vi "Calibration - Config (SubVI).vi"(7 "Action":enum16{"Save", "Load"}(ring)=enum."Load", 8 "error in (no error)":errorcluster, 10 "Path":path, 11 "DS":T2) -> (0 "error out":errorcluster, 3 "DS out":T2={"Timeout"=-1, "LC MC"=[], "TD MC"=[], "Motor Pulse"=0, "Disp M"=[], "LC Unit"=[], "Disp Unit"=[], "TD Unit"=[], "LC Name"=[], "TD Name"=[], "Machine"=enum."Please Select", "Sensor Port"=[]})   [LabVIEW 2019]
uses:
  Controls/Calibration - Data Structure.ctl
  <vilib>/Utility/config.llb/Write Key (String).vi
  <vilib>/Utility/config.llb/Write Key (Double).vi
  <vilib>/Utility/config.llb/Read Key (String).vi
  <vilib>/Utility/config.llb/Read Key (Double).vi
  <vilib>/Utility/config.llb/NI_LVConfig.lvlib
panel:
  in  "Sensor Port":T1(ring)
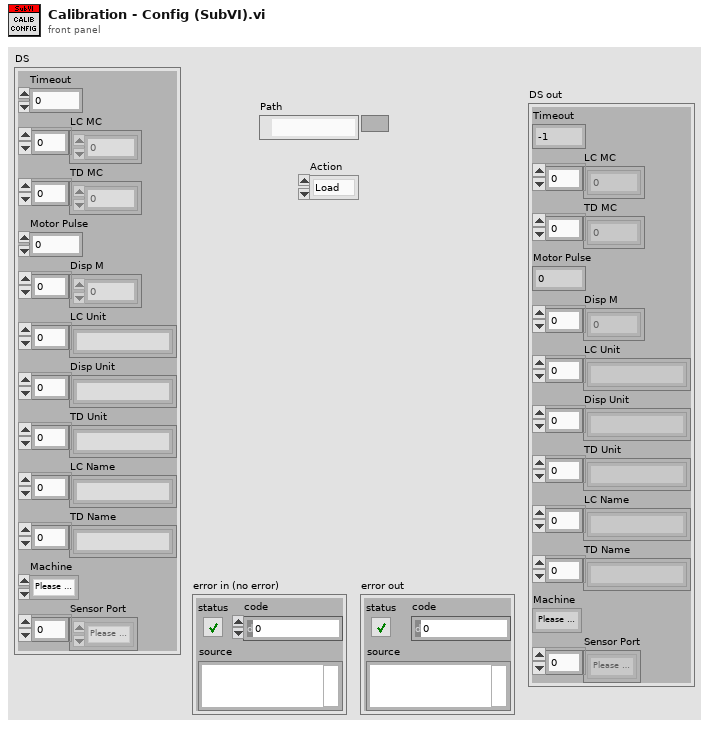
[diagram p1: front panel]
types:
  T1 = enum16{"Please Select", "LC 1", "LC 2", "LC 3", "LC 4", "LC 5", "LC 6", "LC 7", "LC 8", "TD 1", "TD 2", "TD 3", "TD 4", "TD 5", "TD 6", "TD 7", "TD 8", "TD 9", "TD 10", "TD 11", "TD 12"}
  T2 = typedef "Calibration - Data Structure.ctl" = cluster{"Timeout":i32, "LC MC":dbl[], "TD MC":dbl[], "Motor Pulse":u64, "Disp M":dbl[], "LC Unit":string[], "Disp Unit":string[], "TD Unit":string[], "LC Name":string[], "TD Name":string[], "Machine":enum16{"Please Select", "Motor 1", "Motor 2", "Motor 3", "Motor 4", "Motor 5", "Motor 6", "Motor 7", "Motor 8", "Motor 9"}, "Sensor Port":enum16{"Please Select", "LC 1", "LC 2", "LC 3", "LC 4", "LC 5", "LC 6", "LC 7", "LC 8", "TD 1", "TD 2", "TD 3", "TD 4", "TD 5", "TD 6", "TD 7", "TD 8", "TD 9", "TD 10", "TD 11", "TD 12"}[]}
  T3 = typedef "NI_LVConfig.lvlib/Config Data RefNum.ctl" = refnum<k1>
  T4 = enum16{"Please Select", "LC 1", "LC 2", "LC 3", "LC 4", "LC 5", "LC 6", "LC 7", "LC 8", "TD 1", "TD 2", "TD 3", "TD 4", "TD 5", "TD 6", "TD 7", "TD 8", "TD 9", "TD 10", "TD 11", "TD 12"}[]
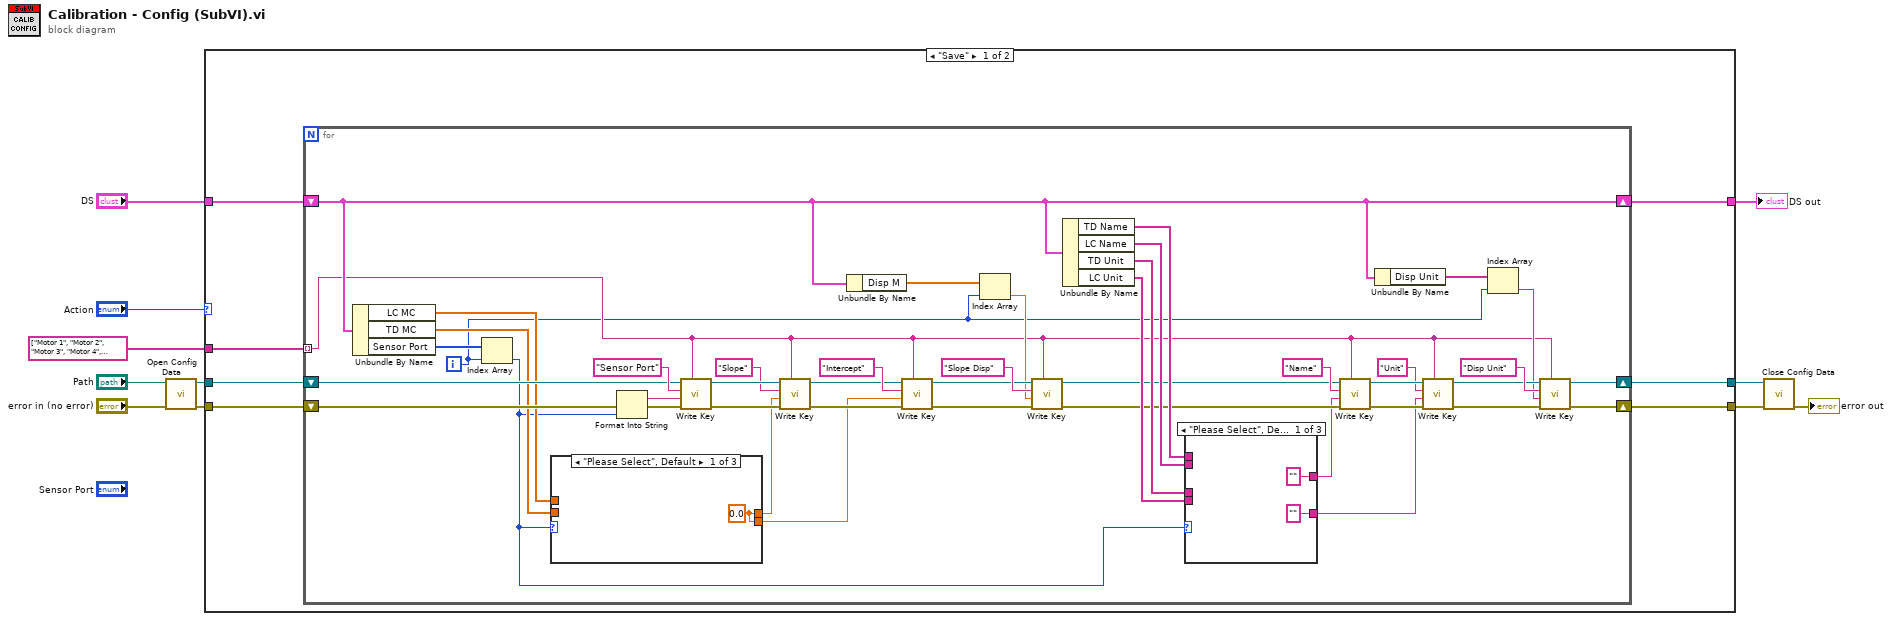
[diagram p0: block diagram]
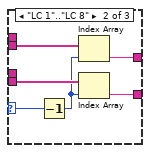
[diagram p2: hidden frame]
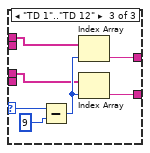
[diagram p3: hidden frame]
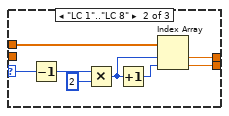
[diagram p4: hidden frame]
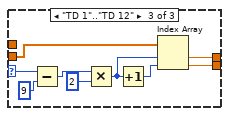
[diagram p5: hidden frame]
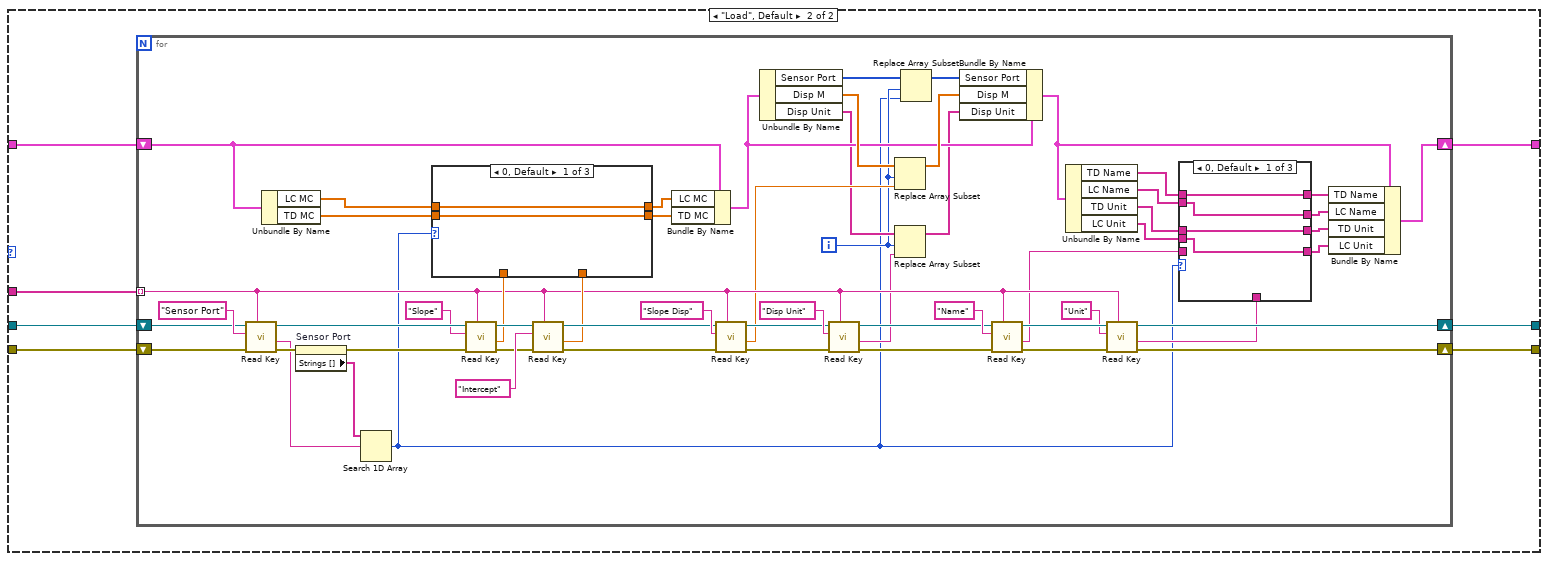
[diagram p6: hidden frame]
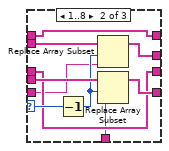
[diagram p7: hidden frame]
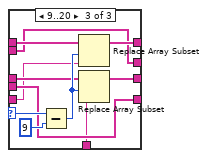
[diagram p8: hidden frame]
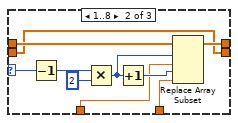
[diagram p9: hidden frame]
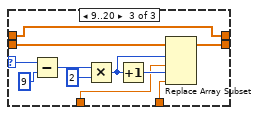
[diagram p10: hidden frame]
diagram:
  n1 = call <vilib>:"Open Config Data.vi"("error in (no error)"="error in (no error)", "configuration file path"="Path") -> ("error out"=w4:errorcluster, "refnum"=w7:T3)  [unwired: 7 in, 1 out]
  n2 = case shown="\"Save\"" "Action" {
    tunnel: "DS" -> [w16 w97]
    tunnel: [w14 w100] -> w9
    tunnel: [w15 w101] -> w8
    tunnel: w7 -> [w17 w102]
    tunnel: w4 -> [w18 w99]
    tunnel: [w13 w98] -> w2
    tunnel: string[] ["Motor 1", "Motor 2", "Motor 3", "Motor 4", "Motor 5", "Motor 6", "Motor 7", "Motor 8", "Motor 9"] ("Strings []") -> [w12 w96]
    frame "Save" {
      n3 = for {
        shift-right: [w22] -> w14
        shift-left: w18 -> [w61]
        shift-right: [w23] -> w15
        shift-left: w17 -> [w58]
        shift-right: [w21] -> w13
        shift-left: w16 -> [w21]
        tunnel: w12 -> [w20] mode=indexing
        i -> [w19]
        n4 = Unbundle By Name(w21) -> ("LC MC"=w50:dbl[], "TD MC"=w51:dbl[], "Sensor Port"=w42:T4)
        n5 = Index Array(array=w42, index=w19) -> (element=w41:T1)
        n6 = case shown="\"Please Select\", Default" w41 {
          selector: w41 -> [_ w85 w90]
          tunnel: w51 -> [_ _ w87]
          tunnel: w50 -> [_ w86 _]
          tunnel: [w78 w80 w92] -> w49
          tunnel: [w78 w79 w91] -> w48
          frame "Please Select", Default {
            w78 = 0.0 ("Numeric")
          }
          frame "LC 1".."LC 8" {
            n7 = Decrement(x=w85) -> (x-1=w83:T1)
            n8 = Multiply(x=w83, y=2) -> (x*y=w81:i32)
            n9 = Increment(x=w81) -> (x+1=w82:i32)
            n10 = Index Array(array=w86, index #1=w81, index #2=w82) -> (element #1=w80:dbl, element #2=w79:dbl)
          }
          frame "TD 1".."TD 12" {
            n11 = Subtract(x=w90, y=9) -> (x-y=w89:i32)
            n12 = Multiply(x=w89, y=2) -> (x*y=w93:i32)
            n13 = Increment(x=w93) -> (x+1=w94:i32)
            n14 = Index Array(array=w87, index #1=w93, index #2=w94) -> (element #1=w92:dbl, element #2=w91:dbl)
          }
        }
        n15 = Format Into String(error in=w61, w41) -> (resulting string=w60:string, error out=w59:errorcluster)  [unwired: 2 in]
        n16 = call-poly <vilib>:"Write Key.vi"("section"=w20, "error in (no error)"=w59, "value"=w60, "key"="Sensor Port" ("section"), "refnum"=w58) -> ("error out"=w57:errorcluster, "refnum out"=w56:T3)  [unwired: 4 in, 1 out]
        n17 = call-poly <vilib>:"Write Key.vi"("section"=w20, "error in (no error)"=w57, "value"=w49, "key"="Slope" ("section"), "refnum"=w56) -> ("error out"=w53:errorcluster, "refnum out"=w52:T3)  [unwired: 4 in, 1 out]
        n18 = Unbundle By Name(w21) -> ("Disp M"=w44:dbl[])
        n19 = call-poly <vilib>:"Write Key.vi"("section"=w20, "error in (no error)"=w53, "value"=w48, "key"="Intercept" ("section"), "refnum"=w52) -> ("error out"=w46:errorcluster, "refnum out"=w45:T3)  [unwired: 4 in, 1 out]
        n20 = Index Array(array=w44, index=w19) -> (element=w43:dbl)
        n21 = call-poly <vilib>:"Write Key.vi"("section"=w20, "error in (no error)"=w46, "value"=w43, "key"="Slope Disp" ("section"), "refnum"=w45) -> ("error out"=w32:errorcluster, "refnum out"=w31:T3)  [unwired: 4 in, 1 out]
        n22 = Unbundle By Name(w21) -> ("TD Name"=w37:string[], "LC Name"=w38:string[], "TD Unit"=w39:string[], "LC Unit"=w40:string[])
        n23 = case shown="\"Please Select\", Default" w41 {
          selector: w41 -> [_ w69 w76]
          tunnel: w40 -> [_ w70 _]
          tunnel: ["" ("String") w68 w77] -> w29
          tunnel: ["" ("String") w66 w73] -> w30
          tunnel: w39 -> [_ _ w72]
          tunnel: w38 -> [_ w65 _]
          tunnel: w37 -> [_ _ w71]
          frame "Please Select", Default {
          }
          frame "LC 1".."LC 8" {
            n24 = Decrement(x=w69) -> (x-1=w67:T1)
            n25 = Index Array(array=w65, index=w67) -> (element=w66:string)
            n26 = Index Array(array=w70, index=w67) -> (element=w68:string)
          }
          frame "TD 1".."TD 12" {
            n27 = Subtract(x=w76, y=9) -> (x-y=w74:i32)
            n28 = Index Array(array=w71, index=w74) -> (element=w73:string)
            n29 = Index Array(array=w72, index=w74) -> (element=w77:string)
          }
        }
        n30 = call-poly <vilib>:"Write Key.vi"("section"=w20, "error in (no error)"=w32, "value"=w30, "key"="Name" ("section"), "refnum"=w31) -> ("error out"=w35:errorcluster, "refnum out"=w36:T3)  [unwired: 4 in, 1 out]
        n31 = Unbundle By Name(w21) -> ("Disp Unit"=w25:string[])
        n32 = call-poly <vilib>:"Write Key.vi"("section"=w20, "error in (no error)"=w35, "value"=w29, "key"="Unit" ("section"), "refnum"=w36) -> ("error out"=w26:errorcluster, "refnum out"=w27:T3)  [unwired: 4 in, 1 out]
        n33 = Index Array(array=w25, index=w19) -> (element=w24:string)
        n34 = call-poly <vilib>:"Write Key.vi"("section"=w20, "error in (no error)"=w26, "value"=w24, "key"="Disp Unit" ("section"), "refnum"=w27) -> ("error out"=w22:errorcluster, "refnum out"=w23:T3)  [unwired: 4 in, 1 out]
      }
    }
    frame "Load", Default {
      n35 = for {
        shift-right: [w121] -> w101
        shift-left: w102 -> [w158]
        shift-right: [w120] -> w100
        shift-left: w99 -> [w144]
        shift-right: [w108] -> w98
        shift-left: w97 -> [w134]
        tunnel: w96 -> [w126] mode=indexing
        i -> [w104]
        n36 = call-poly <vilib>:"Read Key.vi"("section"=w126, "error in (no error)"=w144, "key"="Sensor Port" ("section"), "refnum"=w158) -> ("error out"=w143:errorcluster, "value"=w140:string, "refnum out"=w157:T3)  [unwired: 4 in, 1 out]
        n37 = Unbundle By Name(w134) -> ("LC MC"=w107:dbl[], "TD MC"=w139:dbl[])
        n38 = property on="Sensor Port" class="Enum (strict)"(error in=w143) -> (error out=w142:errorcluster, "Strings []"=w141:string[])  [unwired: 1 in, 1 out]
        n39 = Search 1D Array(1D array=w141, element=w140) -> (index of element=w103:i32)  [unwired: 1 in]
        n40 = call-poly <vilib>:"Read Key.vi"("section"=w126, "error in (no error)"=w142, "key"="Slope" ("section"), "refnum"=w157) -> ("error out"=w154:errorcluster, "value"=w138:dbl, "refnum out"=w153:T3)  [unwired: 4 in, 1 out]
        n41 = call-poly <vilib>:"Read Key.vi"("section"=w126, "error in (no error)"=w154, "key"="Intercept" ("section"), "refnum"=w153) -> ("error out"=w151:errorcluster, "value"=w137:dbl, "refnum out"=w150:T3)  [unwired: 4 in, 1 out]
        n42 = case shown="0, Default" w103 {
          selector: w103 -> [_ w187 w205]
          tunnel: w139 -> [w185 w188 w202]
          tunnel: w107 -> [w186 w196 w197]
          tunnel: w138 -> [_ w190 w200]
          tunnel: w137 -> [_ w191 w199]
          tunnel: [w185 w188 w198] -> w135
          tunnel: [w186 w189 w197] -> w136
          frame 0, Default {
          }
          frame 1..8 {
            n43 = Decrement(x=w187) -> (x-1=w194:i32)
            n44 = Multiply(x=w194, y=2) -> (x*y=w193:i32)
            n45 = Increment(x=w193) -> (x+1=w192:i32)
            n46 = Replace Array Subset(array=w196, new element #1=w190, index #1=w193, new element #2=w191, index #2=w192) -> (w189:dbl[])
          }
          frame 9..20 {
            n47 = Subtract(x=w205, y=9) -> (x-y=w204:i32)
            n48 = Multiply(x=w204, y=2) -> (x*y=w206:i32)
            n49 = Increment(x=w206) -> (x+1=w201:i32)
            n50 = Replace Array Subset(array=w202, new element #1=w200, index #1=w206, new element #2=w199, index #2=w201) -> (w198:dbl[])
          }
        }
        n51 = Bundle By Name(cluster=w134, "LC MC"=w136, "TD MC"=w135) -> (w131:T2)
        n52 = call-poly <vilib>:"Read Key.vi"("section"=w126, "error in (no error)"=w151, "key"="Slope Disp" ("section"), "refnum"=w150) -> ("error out"=w128:errorcluster, "value"=w125:dbl, "refnum out"=w130:T3)  [unwired: 4 in, 1 out]
        n53 = Unbundle By Name(w131) -> ("Sensor Port"=w106:T4, "Disp M"=w133:dbl[], "Disp Unit"=w124:string[])
        n54 = call-poly <vilib>:"Read Key.vi"("section"=w126, "error in (no error)"=w128, "key"="Disp Unit" ("section"), "refnum"=w130) -> ("error out"=w127:errorcluster, "value"=w122:string, "refnum out"=w129:T3)  [unwired: 4 in, 1 out]
        n55 = Replace Array Subset(array=w133, new element=w125, index=w104) -> (w132:dbl[])
        n56 = Replace Array Subset(array=w124, new element=w122, index=w104) -> (w123:string[])
        n57 = Replace Array Subset(array=w106, new element=w103, index=w104) -> (w105:T4)
        n58 = Bundle By Name(cluster=w131, "Sensor Port"=w105, "Disp M"=w132, "Disp Unit"=w123) -> (w109:T2)
        n59 = call-poly <vilib>:"Read Key.vi"("section"=w126, "error in (no error)"=w127, "key"="Name" ("section"), "refnum"=w129) -> ("error out"=w148:errorcluster, "value"=w114:string, "refnum out"=w149:T3)  [unwired: 4 in, 1 out]
        n60 = Unbundle By Name(w109) -> ("TD Name"=w119:string[], "LC Name"=w118:string[], "TD Unit"=w117:string[], "LC Unit"=w116:string[])
        n61 = call-poly <vilib>:"Read Key.vi"("section"=w126, "error in (no error)"=w148, "key"="Unit" ("section"), "refnum"=w149) -> ("error out"=w120:errorcluster, "value"=w115:string, "refnum out"=w121:T3)  [unwired: 4 in, 1 out]
        n62 = case shown="0, Default" w103 {
          selector: w103 -> [_ w172 w184]
          tunnel: w116 -> [w160 w173 w176]
          tunnel: [w160 w171 w176] -> w110
          tunnel: [w162 w169 w177] -> w112
          tunnel: w117 -> [w161 w166 w181]
          tunnel: w118 -> [w162 w168 w177]
          tunnel: w119 -> [w163 w167 w180]
          tunnel: [w163 w167 w179] -> w113
          tunnel: [w161 w166 w178] -> w111
          tunnel: w115 -> [_ w165 w174]
          tunnel: w114 -> [_ w164 w175]
          frame 0, Default {
          }
          frame 1..8 {
            n63 = Decrement(x=w172) -> (x-1=w170:i32)
            n64 = Replace Array Subset(array=w168, new element=w164, index=w170) -> (w169:string[])
            n65 = Replace Array Subset(array=w173, new element=w165, index=w170) -> (w171:string[])
          }
          frame 9..20 {
            n66 = Subtract(x=w184, y=9) -> (x-y=w182:i32)
            n67 = Replace Array Subset(array=w180, new element=w175, index=w182) -> (w179:string[])
            n68 = Replace Array Subset(array=w181, new element=w174, index=w182) -> (w178:string[])
          }
        }
        n69 = Bundle By Name(cluster=w109, "TD Name"=w113, "LC Name"=w112, "TD Unit"=w111, "LC Unit"=w110) -> (w108:T2)
      }
    }
  }
  "DS out" <- w2
  n70 = call <vilib>:"Close Config Data.vi"("error in (no error)"=w9, "refnum"=w8) -> ("error out"=→"error out":errorcluster)  [unwired: 8 in, 1 out]
